vi "Format CSV.vi"(8 "error in (no error)":errorcluster, 9 "delimiter":string=",", 10 "CSV File Input":path, 11 "Original CSV Format":enum16{"Format A", "Format B"}(ring)) -> (0 "error out":errorcluster, 1 "Parcel Length":i32[](array[numeric]), 2 "All Terminal Data":T1(array[cluster]))   [LabVIEW 2017] (continued)
"34:43.4", "34:43.4", "34:43.4", "34:43.5", "34:43.5", "34:43.5", "34:43.6", "34:43.6", "34:43.6", "34:43.7", "34:43.7", "34:43.7", "34:43.8", "34:43.8", "34:43.8", "34:43.9", "34:43.9", "34:43.9", "34:44.0", "34:44.0", "34:44.0", "34:44.1", "34:44.1", "34:44.1", "34:44.2", "34:44.2", "34:44.2", "34:44.3", "34:44.3", "34:44.3", "34:44.4", "34:44.4", "34:44.4", "34:44.5", "34:44.5", "34:44.5", "34:44.6", "34:44.6", "34:44.6", "34:44.7", "34:44.7", "34:44.7", "34:44.8", "34:44.8", "34:44.8", "34:44.9", "34:44.9", "34:44.9", "34:45.0", "34:45.0", "34:45.0", "34:45.1", "34:45.1", "34:45.1", "34:45.2", "34:45.2", "34:45.2", "34:45.3", "34:45.3", "34:45.3", "34:45.4", "34:45.4", "34:45.4", "34:45.5", "34:45.5", "34:45.5", "34:45.6", "34:45.6", "34:45.6", "34:45.7", "34:45.7", "34:45.7", "34:45.8", "34:45.8", "34:45.8", "34:45.9", "34:45.9", "34:45.9", "34:46.0", "34:46.0", "34:46.0", "34:46.1", "34:46.1", "34:46.1", "34:46.2", "34:46.2", "34:46.2", "34:46.3", "34:46.3", "34:46.3", "34:46.4", "34:46.4", "34:46.4", "34:46.5", "34:46.5", "34:46.5", "34:46.6", "34:46.6", "34:46.6", "34:46.7", "34:46.7", "34:46.7", "34:46.8", "34:46.8", "34:46.8", "34:46.9", "34:46.9", "34:46.9", "34:47.0", "34:47.0", "34:47.0", "34:47.1", "34:47.1", "34:47.1", "34:47.2", "34:47.2", "34:47.2", "34:47.3", "34:47.3", "34:47.3", "34:47.4", "34:47.4", "34:47.4", "34:47.5", "34:47.5", "34:47.5", "34:47.6", "34:47.6", "34:47.6", "34:47.7", "34:47.7", "34:47.7", "34:47.8", "34:47.8", "34:47.8", "34:47.9", "34:47.9", "34:47.9", "34:48.0", "34:48.0", "34:48.0", "34:48.1", "34:48.1", "34:48.1", "34:48.2", "34:48.2", "34:48.2", "34:48.3", "34:48.3", "34:48.3", "34:48.4", "34:48.4", "34:48.4", "34:48.5", "34:48.5", "34:48.5", "34:48.6", "34:48.6", "34:48.6", "34:48.7", "34:48.7", "34:48.7", "34:48.8", "34:48.8", "34:48.8", "34:48.9", "34:48.9", "34:48.9", "34:49.0", "34:49.0", "34:49.0", "34:49.1", "34:49.1", "34:49.1", "34:49.2", "34:49.2", "34:49.2", "34:49.3", "34:49.3", "34:49.3", "34:49.4", "34:49.4", "34:49.4", "34:49.5", "34:49.5", "34:49.5", "34:49.6", "34:49.6", "34:49.6", "34:49.7", "34:49.7", "34:49.7", "34:49.8", "34:49.8", "34:49.8", "34:49.9", "34:49.9", "34:49.9", "34:50.0", "34:50.0", "34:50.0", "34:50.1", "34:50.1", "34:50.1", "34:50.2", "34:50.2", "34:50.2", "34:50.3", "34:50.3", "34:50.3", "34:50.4", "34:50.4", "34:50.4", "34:50.5", "34:50.5", "34:50.5", "34:50.6", "34:50.6", "34:50.6", "34:50.7", "34:50.7", "34:50.7", "34:50.8", "34:50.8", "34:50.8", "34:50.9", "34:50.9", "34:50.9", "34:51.0", "34:51.0", "34:51.0", "34:51.1", "34:51.1", "34:51.1", "34:51.2", "34:51.2", "34:51.2", "34:51.3", "34:51.3", "34:51.3", "34:51.4", "34:51.4", "34:51.4", "34:51.5", "34:51.5", "34:51.5", "34:51.6", "34:51.6", "34:51.6", "34:51.7", "34:51.7", "34:51.7", "34:51.8", "34:51.8", "34:51.8", "34:51.9", "34:51.9", "34:51.9", "34:52.0", "34:52.0", "34:52.0", "34:52.1", "34:52.1", "34:52.1", "34:52.2", "34:52.2", "34:52.2", "34:52.3", "34:52.3", "34:52.3", "34:52.4", "34:52.4", "34:52.4", "34:52.5", "34:52.5", "34:52.5", "34:52.6", "34:52.6", "34:52.6", "34:52.7", "34:52.7", "34:52.7", "34:52.8", "34:52.8", "34:52.8", "34:52.9", "34:52.9", "34:52.9", "34:53.0", "34:53.0", "34:53.0", "34:53.1", "34:53.1", "34:53.1", "34:53.2", "34:53.2", "34:53.2", "34:53.3", "34:53.3", "34:53.3", "34:53.4", "34:53.4", "34:53.4", "34:53.5", "34:53.5", "34:53.5", "34:53.6", "34:53.6", "34:53.6", "34:53.7", "34:53.7", "34:53.7", "34:53.8", "34:53.8", "34:53.8", "34:53.9", "34:53.9", "34:53.9", "34:54.0", "34:54.0", "34:54.0", "34:54.1", "34:54.1", "34:54.1", "34:54.2", "34:54.2", "34:54.2", "34:54.3", "34:54.3", "34:54.3", "34:54.4", "34:54.4", "34:54.4", "34:54.5", "34:54.5", "34:54.5", "34:54.6", "34:54.6", "34:54.6", "34:54.7", "34:54.7", "34:54.7", "34:54.8", "34:54.8", "34:54.8", "34:54.9", "34:54.9", "34:54.9", "34:55.0", "34:55.0", "34:55.0", "34:55.1", "34:55.1", "34:55.1", "34:55.2", "34:55.2", "34:55.2", "34:55.3", "34:55.3", "34:55.3", "34:55.4", "34:55.4", "34:55.4", "34:55.5", "34:55.5", "34:55.5", "34:55.6", "34:55.6", "34:55.6", "34:55.7", "34:55.7", "34:55.7", "34:55.8", "34:55.8", "34:55.8", "34:55.9", "34:55.9", "34:55.9", "34:56.0", "34:56.0", "34:56.0", "34:56.1", "34:56.1", "34:56.1", "34:56.2", "34:56.2", "34:56.2", "34:56.3", "34:56.3", "34:56.3", "34:56.4", "34:56.4", "34:56.4", "34:56.5", "34:56.5", "34:56.5", "34:56.6", "34:56.6", "34:56.6", "34:56.7", "34:56.7", "34:56.7", "34:56.8", "34:56.8", "34:56.8", "34:56.9", "34:56.9", "34:56.9", "34:57.0", "34:57.0", "34:57.0", "34:57.1", "34:57.1", "34:57.1", "34:57.2", "34:57.2", "34:57.2", "34:57.3", "34:57.3", "34:57.3", "34:57.4", "34:57.4", "34:57.4", "34:57.5", "34:57.5", "34:57.5", "34:57.6", "34:57.6", "34:57.6", "34:57.7", "34:57.7", "34:57.7", "34:57.8", "34:57.8", "34:57.8", "34:57.9", "34:57.9", "34:57.9", "34:58.0", "34:58.0", "34:58.0", "34:58.1", "34:58.1", "34:58.1", "34:58.2", "34:58.2", "34:58.2", "34:58.3", "34:58.3", "34:58.3", "34:58.4", "34:58.4", "34:58.4", "34:58.5", "34:58.5", "34:58.5", "34:58.6", "34:58.6", "34:58.6", "34:58.7", "34:58.7", "34:58.7", "34:58.8", "34:58.8", "34:58.8", "34:58.9", "34:58.9", "34:58.9", "34:59.0", "34:59.0", "34:59.0", "34:59.1", "34:59.1", "34:59.1", "34:59.2", "34:59.2", "34:59.2", "34:59.3", "34:59.3", "34:59.3", "34:59.4", "34:59.4", "34:59.4", "34:59.5", "34:59.5", "34:59.5", "34:59.6", "34:59.6", "34:59.6", "34:59.7", "34:59.7", "34:59.7", "34:59.8", "34:59.8", "34:59.8", "34:59.9", "34:59.9", "34:59.9", "35:00.0", "35:00.0", "35:00.0", "35:00.1", "35:00.1", "35:00.1", "35:00.2", "35:00.2", "35:00.2", "35:00.3", "35:00.3", "35:00.3", "35:00.4", "35:00.4", "35:00.4", "35:00.5", "35:00.5", "35:00.5", "35:00.6", "35:00.6", "35:00.6", "35:00.7", "35:00.7", "35:00.7", "35:00.8", "35:00.8", "35:00.8", "35:00.9", "35:00.9", "35:00.9", "35:01.0", "35:01.0", "35:01.0", "35:01.1", "35:01.1", "35:01.1", "35:01.2", "35:01.2", "35:01.2", "35:01.3", "35:01.3", "35:01.3", "35:01.4", "35:01.4", "35:01.4", "35:01.5", "35:01.5", "35:01.5", "35:01.6", "35:01.6", "35:01.6", "35:01.7", "35:01.7", "35:01.7", "35:01.8", "35:01.8", "35:01.8", "35:01.9", "35:01.9", "35:01.9", "35:02.0", "35:02.0", "35:02.0", "35:02.1", "35:02.1", "35:02.1", "35:02.2", "35:02.2", "35:02.2", "35:02.3", "35:02.3", "35:02.3", "35:02.4", "35:02.4", "35:02.4", "35:02.5", "35:02.5", "35:02.5", "35:02.6", "35:02.6", "35:02.6", "35:02.7", "35:02.7", "35:02.7", "35:02.8", "35:02.8", "35:02.8", "35:02.9", "35:02.9", "35:02.9", "35:03.0", "35:03.0", "35:03.0", "35:03.1", "35:03.1", "35:03.1", "35:03.2", "35:03.2", "35:03.2", "35:03.3", "35:03.3", "35:03.3", "35:03.4", "35:03.4", "35:03.4", "35:03.5", "35:03.5", "35:03.5", "35:03.6", "35:03.6", "35:03.6", "35:03.7", "35:03.7", "35:03.7", "35:03.8", "35:03.8", "35:03.8", "35:03.9", "35:03.9", "35:03.9", "35:04.0", "35:04.0", "35:04.0", "35:04.1", "35:04.1", "35:04.1", "35:04.2", "35:04.2", "35:04.2", "35:04.3", "35:04.3", "35:04.3", "35:04.4", "35:04.4", "35:04.4", "35:04.5", "35:04.5", "35:04.5", "35:04.6", "35:04.6", "35:04.6", "35:04.7", "35:04.7", "35:04.7", "35:04.8", "35:04.8", "35:04.8", "35:04.9", "35:04.9", "35:04.9", "35:05.0", "35:05.0", "35:05.0", "35:05.1", "35:05.1", "35:05.1", "35:05.2", "35:05.2", "35:05.2", "35:05.3", "35:05.3", "35:05.3", "35:05.4", "35:05.4", "35:05.4", "35:05.5", "35:05.5", "35:05.5", "35:05.6", "35:05.6", "35:05.6", "35:05.7", "35:05.7", "35:05.7", "35:05.8", "35:05.8", "35:05.8", "35:05.9", "35:05.9", "35:05.9", "35:06.0", "35:06.0", "35:06.0", "35:06.1", "35:06.1", "35:06.1", "35:06.2", "35:06.2", "35:06.2", "35:06.3", "35:06.3", "35:06.3", "35:06.4", "35:06.4", "35:06.4", "35:06.5", "35:06.5", "35:06.5", "35:06.6", "35:06.6", "35:06.6", "35:06.7", "35:06.7", "35:06.7", "35:06.8", "35:06.8", "35:06.8", "35:06.9", "35:06.9", "35:06.9", "35:07.0", "35:07.0", "35:07.0", "35:07.1", "35:07.1", "35:07.1", "35:07.2", "35:07.2", "35:07.2", "35:07.3", "35:07.3", "35:07.3", "35:07.4", "35:07.4", "35:07.4", "35:07.5", "35:07.5", "35:07.5", "35:07.6", "35:07.6", "35:07.6", "35:07.7", "35:07.7", "35:07.7", "35:07.8", "35:07.8", "35:07.8", "35:07.9", "35:07.9", "35:07.9", "35:08.0", "35:08.0", "35:08.0", "35:08.1", "35:08.1", "35:08.1", "35:08.2", "35:08.2", "35:08.2", "35:08.3", "35:08.3", "35:08.3", "35:08.4", "35:08.4", "35:08.4", "35:08.5", "35:08.5", "35:08.5", "35:08.6", "35:08.6", "35:08.6", "35:08.7", "35:08.7", "35:08.7", "35:08.8", "35:08.8", "35:08.8", "35:08.9", "35:08.9", "35:08.9", "35:09.0", "35:09.0", "35:09.0", "35:09.1", "35:09.1", "35:09.1", "35:09.2", "35:09.2", "35:09.2", "35:09.3", "35:09.3", "35:09.3", "35:09.4", "35:09.4", "35:09.4", "35:09.5", "35:09.5", "35:09.5", "35:09.6", "35:09.6", "35:09.6", "35:09.7", "35:09.7", "35:09.7", "35:09.8", "35:09.8", "35:09.8", "35:09.9", "35:09.9", "35:09.9", "35:10.0", "35:10.0", "35:10.0", "35:10.1", "35:10.1", "35:10.1", "35:10.2", "35:10.2", "35:10.2", "35:10.3", "35:10.3", "35:10.3", "35:10.4", "35:10.4", "35:10.4", "35:10.5", "35:10.5", "35:10.5", "35:10.6", "35:10.6", "35:10.6", "35:10.7", "35:10.7", "35:10.7", "35:10.8", "35:10.8", "35:10.8", "35:10.9", "35:10.9", "35:10.9", "35:11.0", "35:11.0", "35:11.0", "35:11.1", "35:11.1", "35:11.1", "35:11.2", "35:11.2", "35:11.2", "35:11.3", "35:11.3", "35:11.3", "35:11.4", "35:11.4", "35:11.4", "35:11.5", "35:11.5", "35:11.5", "35:11.6", "35:11.6", "35:11.6", "35:11.7", "35:11.7", "35:11.7", "35:11.8", "35:11.8", "35:11.8", "35:11.9", "35:11.9", "35:11.9", "35:12.0", "35:12.0", "35:12.0", "35:12.1", "35:12.1", "35:12.1", "35:12.2", "35:12.2", "35:12.2", "35:12.3", "35:12.3", "35:12.3", "35:12.4", "35:12.4", "35:12.4", "35:12.5", "35:12.5", "35:12.5", "35:12.6", "35:12.6", "35:12.6", "35:12.7", "35:12.7", "35:12.7", "35:12.8", "35:12.8", "35:12.8", "35:12.9", "35:12.9", "35:12.9", "35:13.0", "35:13.0", "35:13.0", "35:13.1", "35:13.1", "35:13.1", "35:13.2", "35:13.2", "35:13.2", "35:13.3", "35:13.3", "35:13.3", "35:13.4", "35:13.4", "35:13.4", "35:13.5", "35:13.5", "35:13.5", "35:13.6", "35:13.6", "35:13.6", "35:13.7", "35:13.7", "35:13.7", "35:13.8", "35:13.8", "35:13.8", "35:13.9", "35:13.9", "35:13.9", "35:14.0", "35:14.0", "35:14.0", "35:14.1", "35:14.1", "35:14.1", "35:14.2", "35:14.2", "35:14.2", "35:14.3", "35:14.3", "35:14.3", "35:14.4", "35:14.4", "35:14.4", "35:14.5", "35:14.5", "35:14.5", "35:14.6", "35:14.6", "35:14.6", "35:14.7", "35:14.7", "35:14.7", "35:14.8", "35:14.8", "35:14.8", "35:14.9", "35:14.9", "35:14.9", "35:15.0", "35:15.0", "35:15.0", "35:15.1", "35:15.1", "35:15.1", "35:15.2", "35:15.2", "35:15.2", "35:15.3", "35:15.3", "35:15.3", "35:15.4", "35:15.4", "35:15.4", "35:15.5", "35:15.5", "35:15.5", "35:15.6", "35:15.6", "35:15.6", "35:15.7", "35:15.7", "35:15.7", "35:15.8", "35:15.8", "35:15.8", "35:15.9", "35:15.9", "35:15.9", "35:16.0", "35:16.0", "35:16.0", "35:16.1", "35:16.1", "35:16.1", "35:16.2", "35:16.2", "35:16.2", "35:16.3", "35:16.3", "35:16.3", "35:16.4", "35:16.4", "35:16.4", "35:16.5", "35:16.5", "35:16.5", "35:16.6", "35:16.6", "35:16.6", "35:16.7", "35:16.7", "35:16.7", "35:16.8", "35:16.8", "35:16.8", "35:16.9", "35:16.9", "35:16.9", "35:17.0", "35:17.0", "35:17.0", "35:17.1", "35:17.1", "35:17.1", "35:17.2", "35:17.2", "35:17.2", "35:17.3", "35:17.3", "35:17.3", "35:17.4", "35:17.4", "35:17.4", "35:17.5", "35:17.5", "35:17.5", "35:17.6", "35:17.6", "35:17.6", "35:17.7", "35:17.7", "35:17.7", "35:17.8", "35:17.8", "35:17.8", "35:17.9", "35:17.9", "35:17.9", "35:18.0", "35:18.0", "35:18.0", "35:18.1", "35:18.1", "35:18.1", "35:18.2", "35:18.2", "35:18.2", "35:18.3", "35:18.3", "35:18.3", "35:18.4", "35:18.4", "35:18.4", "35:18.5", "35:18.5", "35:18.5", "35:18.6", "35:18.6", "35:18.6", "35:18.7", "35:18.7", "35:18.7", "35:18.8", "35:18.8", "35:18.8", "35:18.9", "35:18.9", "35:18.9", "35:19.0", "35:19.0", "35:19.0", "35:19.1", "35:19.1", "35:19.1", "35:19.2", "35:19.2", "35:19.2", "35:19.3", "35:19.3", "35:19.3", "35:19.4", "35:19.4", "35:19.4", "35:19.5", "35:19.5", "35:19.5", "35:19.6", "35:19.6", "35:19.6", "35:19.7", "35:19.7", "35:19.7", "35:19.8", "35:19.8", "35:19.8", "35:19.9", "35:19.9", "35:19.9", "35:20.0", "35:20.0", "35:20.0", "35:20.1", "35:20.1", "35:20.1", "35:20.2", "35:20.2", "35:20.2", "35:20.3", "35:20.3", "35:20.3", "35:20.4", "35:20.4", "35:20.4", "35:20.5", "35:20.5", "35:20.5", "35:20.6", "35:20.6", "35:20.6", "35:20.7", "35:20.7", "35:20.7", "35:20.8", "35:20.8", "35:20.8", "35:20.9", "35:20.9", "35:20.9", "35:21.0", "35:21.0", "35:21.0", "35:21.1", "35:21.1", "35:21.1", "35:21.2", "35:21.2", "35:21.2", "35:21.3", "35:21.3", "35:21.3", "35:21.4", "35:21.4", "35:21.4", "35:21.5", "35:21.5", "35:21.5", "35:21.6", "35:21.6", "35:21.6", "35:21.7", "35:21.7", "35:21.7", "35:21.8", "35:21.8", "35:21.8", "35:21.9", "35:21.9", "35:21.9", "35:22.0", "35:22.0", "35:22.0", "35:22.1", "35:22.1", "35:22.1", "35:22.2", "35:22.2", "35:22.2", "35:22.3", "35:22.3", "35:22.3", "35:22.4", "35:22.4", "35:22.4", "35:22.5", "35:22.5", "35:22.5", "35:22.6", "35:22.6", "35:22.6", "35:22.7", "35:22.7", "35:22.7", "35:22.8", "35:22.8", "35:22.8", "35:22.9", "35:22.9", "35:22.9", "35:23.0", "35:23.0", "35:23.0", "35:23.1", "35:23.1", "35:23.1", "35:23.2", "35:23.2", "35:23.2", "35:23.3", "35:23.3", "35:23.3", "35:23.4", "35:23.4", "35:23.4", "35:23.5", "35:23.5", "35:23.5", "35:23.6", "35:23.6", "35:23.6", "35:23.7", "35:23.7", "35:23.7", "35:23.8", "35:23.8", "35:23.8", "35:23.9", "35:23.9", "35:23.9", "35:24.0", "35:24.0", "35:24.0", "35:24.1", "35:24.1", "35:24.1", "35:24.2", "35:24.2", "35:24.2", "35:24.3", "35:24.3", "35:24.3", "35:24.4", "35:24.4", "35:24.4", "35:24.5", "35:24.5", "35:24.5", "35:24.6", "35:24.6", "35:24.6", "35:24.7", "35:24.7", "35:24.7", "35:24.8", "35:24.8", "35:24.8", "35:24.9", "35:24.9", "35:24.9", "35:25.0", "35:25.0", "35:25.0", "35:25.1", "35:25.1", "35:25.1", "35:25.2", "35:25.2", "35:25.2", "35:25.3", "35:25.3", "35:25.3", "35:25.4", "35:25.4", "35:25.4", "35:25.5", "35:25.5", "35:25.5", "35:25.6", "35:25.6", "35:25.6", "35:25.7", "35:25.7", "35:25.7", "35:25.8", "35:25.8", "35:25.8", "35:25.9", "35:25.9", "35:25.9", "35:26.0", "35:26.0", "35:26.0", "35:26.1", "35:26.1", "35:26.1", "35:26.2", "35:26.2", "35:26.2", "35:26.3", "35:26.3", "35:26.3", "35:26.4", "35:26.4", "35:26.4", "35:26.5", "35:26.5", "35:26.5", "35:26.6", "35:26.6", "35:26.6", "35:26.7", "35:26.7", "35:26.7", "35:26.8", "35:26.8", "35:26.8", "35:26.9", "35:26.9", "35:26.9", "35:27.0", "35:27.0", "35:27.0", "35:27.1", "35:27.1", "35:27.1", "35:27.2", "35:27.2", "35:27.2", "35:27.3", "35:27.3", "35:27.3", "35:27.4", "35:27.4", "35:27.4", "35:27.5", "35:27.5", "35:27.5", "35:27.6", "35:27.6", "35:27.6", "35:27.7", "35:27.7", "35:27.7", "35:27.8", "35:27.8", "35:27.8", "35:27.9", "35:27.9", "35:27.9", "35:28.0", "35:28.0", "35:28.0", "35:28.1", "35:28.1", "35:28.1", "35:28.2", "35:28.2", "35:28.2", "35:28.3", "35:28.3", "35:28.3", "35:28.4", "35:28.4", "35:28.4", "35:28.5", "35:28.5", "35:28.5", "35:28.6", "35:28.6", "35:28.6", "35:28.7", "35:28.7", "35:28.7", "35:28.8", "35:28.8", "35:28.8", "35:28.9", "35:28.9", "35:28.9", "35:29.0", "35:29.0", "35:29.0", "35:29.1", "35:29.1", "35:29.1", "35:29.2", "35:29.2", "35:29.2", "35:29.3", "35:29.3", "35:29.3", "35:29.4", "35:29.4", "35:29.4", "35:29.5", "35:29.5", "35:29.5", "35:29.6", "35:29.6", "35:29.6", "35:29.7", "35:29.7", "35:29.7", "35:29.8", "35:29.8", "35:29.8", "35:29.9", "35:29.9", "35:29.9", "35:30.0", "35:30.0", "35:30.0", "35:30.1", "35:30.1", "35:30.1", "35:30.2", "35:30.2", "35:30.2", "35:30.3", "35:30.3", "35:30.3", "35:30.4", "35:30.4", "35:30.4", "35:30.5", "35:30.5", "35:30.5", "35:30.6", "35:30.6", "35:30.6", "35:30.7", "35:30.7", "35:30.7", "35:30.8", "35:30.8", "35:30.8", "35:30.9", "35:30.9", "35:30.9", "35:31.0", "35:31.0", "35:31.0", "35:31.1", "35:31.1", "35:31.1", "35:31.2", "35:31.2", "35:31.2", "35:31.3", "35:31.3", "35:31.3", "35:31.4", "35:31.4", "35:31.4", "35:31.5", "35:31.5", "35:31.5", "35:31.6", "35:31.6", "35:31.6", "35:31.7", "35:31.7", "35:31.7", "35:31.8", "35:31.8", "35:31.8", "35:31.9", "35:31.9", "35:31.9", "35:32.0", "35:32.0", "35:32.0", "35:32.1", "35:32.1", "35:32.1", "35:32.2", "35:32.2", "35:32.2", "35:32.3", "35:32.3", "35:32.3", "35:32.4", "35:32.4", "35:32.4", "35:32.5", "35:32.5", "35:32.5", "35:32.6", "35:32.6", "35:32.6", "35:32.7", "35:32.7", "35:32.7", "35:32.8", "35:32.8", "35:32.8", "35:32.9", "35:32.9", "35:32.9", "35:33.0", "35:33.0", "35:33.0", "35:33.1", "35:33.1", "35:33.1", "35:33.2", "35:33.2", "35:33.2", "35:33.3", "35:33.3", "35:33.3", "35:33.4", "35:33.4", "35:33.4", "35:33.5", "35:33.5", "35:33.5", "35:33.6", "35:33.6", "35:33.6", "35:33.7", "35:33.7", "35:33.7", "35:33.8", "35:33.8", "35:33.8", "35:33.9", "35:33.9", "35:33.9", "35:34.0", "35:34.0", "35:34.0", "35:34.1", "35:34.1", "35:34.1", "35:34.2", "35:34.2", "35:34.2", "35:34.3", "35:34.3", "35:34.3", "35:34.4", "35:34.4", "35:34.4", "35:34.5", "35:34.5", "35:34.5", "35:34.6", "35:34.6", "35:34.6", "35:34.7", "35:34.7", "35:34.7", "35:34.8", "35:34.8", "35:34.8", "35:34.9", "35:34.9", "35:34.9", "35:35.0", "35:35.0", "35:35.0", "35:35.1", "35:35.1", "35:35.1", "35:35.2", "35:35.2", "35:35.2", "35:35.3", "35:35.3", "35:35.3", "35:35.4", "35:35.4", "35:35.4", "35:35.5", "35:35.5", "35:35.5", "35:35.6", "35:35.6", "35:35.6", "35:35.7", "35:35.7", "35:35.7", "35:35.8", "35:35.8", "35:35.8", "35:35.9", "35:35.9", "35:35.9", "35:36.0", "35:36.0", "35:36.0", "35:36.1", "35:36.1", "35:36.1", "35:36.2", "35:36.2", "35:36.2", "35:36.3", "35:36.3", "35:36.3", "35:36.4", "35:36.4", "35:36.4", "35:36.5", "35:36.5", "35:36.5", "35:36.6", "35:36.6", "35:36.6", "35:36.7", "35:36.7", "35:36.7", "35:36.8", "35:36.8", "35:36.8", "35:36.9", "35:36.9", "35:36.9", "35:37.0", "35:37.0", "35:37.0", "35:37.1", "35:37.1", "35:37.1", "35:37.2", "35:37.2", "35:37.2", "35:37.3", "35:37.3", "35:37.3", "35:37.4", "35:37.4", "35:37.4", "35:37.5", "35:37.5", "35:37.5", "35:37.6", "35:37.6", "35:37.6", "35:37.7", "35:37.7", "35:37.7", "35:37.8", "35:37.8", "35:37.8", "35:37.9", "35:37.9", "35:37.9", "35:38.0", "35:38.0", "35:38.0", "35:38.1", "35:38.1", "35:38.1", "35:38.2", "35:38.2", "35:38.2", "35:38.3", "35:38.3", "35:38.3", "35:38.4", "35:38.4", "35:38.4", "35:38.5", "35:38.5", "35:38.5", "35:38.6", "35:38.6", "35:38.6", "35:38.7", "35:38.7", "35:38.7", "35:38.8", "35:38.8", "35:38.8", "35:38.9", "35:38.9", "35:38.9", "35:39.0", "35:39.0", "35:39.0", "35:39.1", "35:39.1", "35:39.1", "35:39.2", "35:39.2", "35:39.2", "35:39.3", "35:39.3", "35:39.3", "35:39.4", "35:39.4", "35:39.4", "35:39.5", "35:39.5", "35:39.5", "35:39.6", "35:39.6", "35:39.6", "35:39.7", "35:39.7", "35:39.7", "35:39.8", "35:39.8", "35:39.8", "35:39.9", "35:39.9", "35:39.9", "35:40.0", "35:40.0", "35:40.0", "35:40.1", "35:40.1", "35:40.1", "35:40.2", "35:40.2", "35:40.2", "35:40.3", "35:40.3", "35:40.3", "35:40.4", "35:40.4", "35:40.4", "35:40.5", "35:40.5", "35:40.5", "35:40.6", "35:40.6", "35:40.6", "35:40.7", "35:40.7", "35:40.7", "35:40.8", "35:40.8", "35:40.8", "35:40.9", "35:40.9", "35:40.9", "35:41.0", "35:41.0", "35:41.0", "35:41.1", "35:41.1", "35:41.1", "35:41.2", "35:41.2", "35:41.2", "35:41.3", "35:41.3", "35:41.3", "35:41.4", "35:41.4", "35:41.4", "35:41.5", "35:41.5", "35:41.5", "35:41.6", "35:41.6", "35:41.6", "35:41.7", "35:41.7", "35:41.7", "35:41.8", "35:41.8", "35:41.8", "35:41.9", "35:41.9", "35:41.9", "35:42.0", "35:42.0", "35:42.0", "35:42.1", "35:42.1", "35:42.1", "35:42.2", "35:42.2", "35:42.2", "35:42.3", "35:42.3", "35:42.3", "35:42.4", "35:42.4", "35:42.4", "35:42.5", "35:42.5", "35:42.5", "35:42.6", "35:42.6", "35:42.6", "35:42.7", "35:42.7", "35:42.7", "35:42.8", "35:42.8", "35:42.8", "35:42.9", "35:42.9", "35:42.9", "35:43.0", "35:43.0", "35:43.0", "35:43.1", "35:43.1", "35:43.1", "35:43.2", "35:43.2", "35:43.2", "35:43.3", "35:43.3", "35:43.3", "35:43.4", "35:43.4", "35:43.4", "35:43.5", "35:43.5", "35:43.5", "35:43.6", "35:43.6", "35:43.6", "35:43.7", "35:43.7", "35:43.7", "35:43.8", "35:43.8", "35:43.8", "35:43.9", "35:43.9", "35:43.9", "35:44.0", "35:44.0", "35:44.0", "35:44.1", "35:44.1", "35:44.1", "35:44.2", "35:44.2", "35:44.2", "35:44.3", "35:44.3", "35:44.3", "35:44.4", "35:44.4", "35:44.4", "35:44.5", "35:44.5", "35:44.5", "35:44.6", "35:44.6", "35:44.6", "35:44.7", "35:44.7", "35:44.7", "35:44.8", "35:44.8", "35:44.8", "35:44.9", "35:44.9", "35:44.9", "35:45.0", "35:45.0", "35:45.0", "35:45.1", "35:45.1", "35:45.1", "35:45.2", "35:45.2", "35:45.2", "35:45.3", "35:45.3", "35:45.3", "35:45.4", "35:45.4", "35:45.4", "35:45.5", "35:45.5", "35:45.5", "35:45.6", "35:45.6", "35:45.6", "35:45.7", "35:45.7", "35:45.7", "35:45.8", "35:45.8", "35:45.8", "35:45.9", "35:45.9", "35:45.9", "35:46.0", "35:46.0", "35:46.0", "35:46.1", "35:46.1", "35:46.1", "35:46.2", "35:46.2", "35:46.2", "35:46.3", "35:46.3", "35:46.3", "35:46.4", "35:46.4", "35:46.4", "35:46.5", "35:46.5", "35:46.5", "35:46.6", "35:46.6", "35:46.6", "35:46.7", "35:46.7", "35:46.7", "35:46.8", "35:46.8", "35:46.8", "35:46.9", "35:46.9", "35:46.9", "35:47.0", "35:47.0", "35:47.0", "35:47.1", "35:47.1", "35:47.1", "35:47.2", "35:47.2", "35:47.2", "35:47.3", "35:47.3", "35:47.3", "35:47.4", "35:47.4", "35:47.4", "35:47.5", "35:47.5", "35:47.5", "35:47.6", "35:47.6", "35:47.6", "35:47.7", "35:47.7", "35:47.7", "35:47.8", "35:47.8", "35:47.8", "35:47.9", "35:47.9", "35:47.9", "35:48.0", "35:48.0", "35:48.0", "35:48.1", "35:48.1", "35:48.1", "35:48.2", "35:48.2", "35:48.2", "35:48.3", "35:48.3", "35:48.3", "35:48.4", "35:48.4", "35:48.4", "35:48.5", "35:48.5", "35:48.5", "35:48.6", "35:48.6", "35:48.6", "35:48.7", "35:48.7", "35:48.7", "35:48.8", "35:48.8", "35:48.8", "35:48.9", "35:48.9", "35:48.9", "35:49.0", "35:49.0", "35:49.0", "35:49.1", "35:49.1", "35:49.1", "35:49.2", "35:49.2", "35:49.2", "35:49.3", "35:49.3", "35:49.3", "35:49.4", "35:49.4", "35:49.4", "35:49.5", "35:49.5", "35:49.5", "35:49.6", "35:49.6", "35:49.6", "35:49.7", "35:49.7", "35:49.7", "35:49.8", "35:49.8", "35:49.8", "35:49.9", "35:49.9", "35:49.9", "35:50.0", "35:50.0", "35:50.0", "35:50.1", "35:50.1", "35:50.1", "35:50.2", "35:50.2", "35:50.2", "35:50.3", "35:50.3", "35:50.3", "35:50.4", "35:50.4", "35:50.4", "35:50.5", "35:50.5", "35:50.5", "35:50.6", "35:50.6", "35:50.6", "35:50.7", "35:50.7", "35:50.7", "35:50.8", "35:50.8", "35:50.8", "35:50.9", "35:50.9", "35:50.9", "35:51.0", "35:51.0", "35:51.0", "35:51.1", "35:51.1", "35:51.1", "35:51.2", "35:51.2", "35:51.2", "35:51.3", "35:51.3", "35:51.3", "35:51.4", "35:51.4", "35:51.4", "35:51.5", "35:51.5", "35:51.5", "35:51.6", "35:51.6", "35:51.6", "35:51.7", "35:51.7", "35:51.7", "35:51.8", "35:51.8", "35:51.8", "35:51.9", "35:51.9", "35:51.9", "35:52.0", "35:52.0", "35:52.0", "35:52.1", "35:52.1", "35:52.1", "35:52.2", "35:52.2", "35:52.2", "35:52.3", "35:52.3", "35:52.3", "35:52.4", "35:52.4", "35:52.4", "35:52.5", "35:52.5", "35:52.5", "35:52.6", "35:52.6", "35:52.6", "35:52.7", "35:52.7", "35:52.7", "35:52.8", "35:52.8", "35:52.8", "35:52.9", "35:52.9", "35:52.9", "35:53.0", "35:53.0", "35:53.0", "35:53.1", "35:53.1", "35:53.1", "35:53.2", "35:53.2", "35:53.2", "35:53.3", "35:53.3", "35:53.3", "35:53.4", "35:53.4", "35:53.4", "35:53.5", "35:53.5", "35:53.5", "35:53.6", "35:53.6", "35:53.6", "35:53.7", "35:53.7", "35:53.7", "35:53.8", "35:53.8", "35:53.8", "35:53.9", "35:53.9", "35:53.9", "35:54.0", "35:54.0", "35:54.0", "35:54.1", "35:54.1", "35:54.1", "35:54.2", "35:54.2", "35:54.2", "35:54.3", "35:54.3", "35:54.3", "35:54.4", "35:54.4", "35:54.4", "35:54.5", "35:54.5", "35:54.5", "35:54.6", "35:54.6", "35:54.6", "35:54.7", "35:54.7", "35:54.7", "35:54.8", "35:54.8", "35:54.8", "35:54.9", "35:54.9", "35:54.9", "35:55.0", "35:55.0", "35:55.0", "35:55.1", "35:55.1", "35:55.1", "35:55.2", "35:55.2", "35:55.2", "35:55.3", "35:55.3", "35:55.3", "35:55.4", "35:55.4", "35:55.4", "35:55.5", "35:55.5", "35:55.5", "35:55.6", "35:55.6", "35:55.6", "35:55.7", "35:55.7", "35:55.7", "35:55.8", "35:55.8", "35:55.8", "35:55.9", "35:55.9", "35:55.9", "35:56.0", "35:56.0", "35:56.0", "35:56.1", "35:56.1", "35:56.1", "35:56.2", "35:56.2", "35:56.2", "35:56.3", "35:56.3", "35:56.3", "35:56.4", "35:56.4", "35:56.4", "35:56.5", "35:56.5", "35:56.5", "35:56.6", "35:56.6", "35:56.6", "35:56.7", "35:56.7", "35:56.7", "35:56.8", "35:56.8", "35:56.8", "35:56.9", "35:56.9", "35:56.9", "35:57.0", "35:57.0", "35:57.0", "35:57.1", "35:57.1", "35:57.1", "35:57.2", "35:57.2", "35:57.2", "35:57.3", "35:57.3", "35:57.3", "35:57.4", "35:57.4", "35:57.4", "35:57.5", "35:57.5", "35:57.5", "35:57.6", "35:57.6", "35:57.6", "35:57.7", "35:57.7", "35:57.7", "35:57.8", "35:57.8", "35:57.8", "35:57.9", "35:57.9", "35:57.9", "35:58.0", "35:58.0", "35:58.0", "35:58.1", "35:58.1", "35:58.1", "35:58.2", "35:58.2", "35:58.2", "35:58.3", "35:58.3", "35:58.3", "35:58.4", "35:58.4", "35:58.4", "35:58.5", "35:58.5", "35:58.5", "35:58.6", "35:58.6", "35:58.6", "35:58.7", "35:58.7", "35:58.7", "35:58.8", "35:58.8", "35:58.8", "35:58.9", "35:58.9", "35:58.9", "35:59.0", "35:59.0", "35:59.0", "35:59.1", "35:59.1", "35:59.1", "35:59.2", "35:59.2", "35:59.2", "35:59.3", "35:59.3", "35:59.3", "35:59.4", "35:59.4", "35:59.4", "35:59.5", "35:59.5", "35:59.5", "35:59.6", "35:59.6", "35:59.6", "35:59.7", "35:59.7", "35:59.7", "35:59.8", "35:59.8", "35:59.8", "35:59.9", "35:59.9", "35:59.9", "36:00.0", "36:00.0", "36:00.0", "36:00.1", "36:00.1", "36:00.1", "36:00.2", "36:00.2", "36:00.2", "36:00.3", "36:00.3", "36:00.3", "36:00.4", "36:00.4", "36:00.4", "36:00.5", "36:00.5", "36:00.5", "36:00.6", "36:00.6", "36:00.6", "36:00.7", "36:00.7", "36:00.7", "36:00.8", "36:00.8", "36:00.8", "36:00.9", "36:00.9", "36:00.9", "36:01.0", "36:01.0", "36:01.0", "36:01.1", "36:01.1", "36:01.1", "36:01.2", "36:01.2", "36:01.2", "36:01.3", "36:01.3", "36:01.3", "36:01.4", "36:01.4", "36:01.4", "36:01.5", "36:01.5", "36:01.5", "36:01.6", "36:01.6", "36:01.6", "36:01.7", "36:01.7", "36:01.7", "36:01.8", "36:01.8", "36:01.8", "36:01.9", "36:01.9", "36:01.9", "36:02.0", "36:02.0", "36:02.0", "36:02.1", "36:02.1", "36:02.1", "36:02.2", "36:02.2", "36:02.2", "36:02.3", "36:02.3", "36:02.3", "36:02.4", "36:02.4", "36:02.4", "36:02.5", "36:02.5", "36:02.5", "36:02.6", "36:02.6", "36:02.6", "36:02.7", "36:02.7", "36:02.7", "36:02.8", "36:02.8", "36:02.8", "36:02.9", "36:02.9", "36:02.9", "36:03.0", "36:03.0", "36:03.0", "36:03.1", "36:03.1", "36:03.1", "36:03.2", "36:03.2", "36:03.2", "36:03.3", "36:03.3", "36:03.3", "36:03.4", "36:03.4", "36:03.4", "36:03.5", "36:03.5", "36:03.5", "36:03.6", "36:03.6", "36:03.6", "36:03.7", "36:03.7", "36:03.7", "36:03.8", "36:03.8", "36:03.8", "36:03.9", "36:03.9", "36:03.9", "36:04.0", "36:04.0", "36:04.0", "36:04.1", "36:04.1", "36:04.1", "36:04.2", "36:04.2", "36:04.2", "36:04.3", "36:04.3", "36:04.3", "36:04.4", "36:04.4", "36:04.4", "36:04.5", "36:04.5", "36:04.5", "36:04.6", "36:04.6", "36:04.6", "36:04.7", "36:04.7", "36:04.7", "36:04.8", "36:04.8", "36:04.8", "36:04.9", "36:04.9", "36:04.9", "36:05.0", "36:05.0", "36:05.0", "36:05.1", "36:05.1", "36:05.1", "36:05.2", "36:05.2", "36:05.2", "36:05.3", "36:05.3", "36:05.3", "36:05.4", "36:05.4", "36:05.4", "36:05.5", "36:05.5", "36:05.5", "36:05.6", "36:05.6", "36:05.6", "36:05.7", "36:05.7", "36:05.7", "36:05.8", "36:05.8", "36:05.8", "36:05.9", "36:05.9", "36:05.9", "36:06.0", "36:06.0", "36:06.0", "36:06.1", "36:06.1", "36:06.1", "36:06.2", "36:06.2", "36:06.2", "36:06.3", "36:06.3", "36:06.3", "36:06.4", "36:06.4", "36:06.4", "36:06.5", "36:06.5", "36:06.5", "36:06.6", "36:06.6", "36:06.6", "36:06.7", "36:06.7", "36:06.7", "36:06.8", "36:06.8", "36:06.8", "36:06.9", "36:06.9", "36:06.9", "36:07.0", "36:07.0", "36:07.0", "36:07.1", "36:07.1", "36:07.1", "36:07.2", "36:07.2", "36:07.2", "36:07.3", "36:07.3", "36:07.3", "36:07.4", "36:07.4", "36:07.4", "36:07.5", "36:07.5", "36:07.5", "36:07.6", "36:07.6", "36:07.6", "36:07.7", "36:07.7", "36:07.7", "36:07.8", "36:07.8", "36:07.8", "36:07.9", "36:07.9", "36:07.9", "36:08.0", "36:08.0", "36:08.0", "36:08.1", "36:08.1", "36:08.1", "36:08.2", "36:08.2", "36:08.2", "36:08.3", "36:08.3", "36:08.3", "36:08.4", "36:08.4", "36:08.4", "36:08.5", "36:08.5", "36:08.5", "36:08.6", "36:08.6", "36:08.6", "36:08.7", "36:08.7", "36:08.7", "36:08.8", "36:08.8", "36:08.8", "36:08.9", "36:08.9", "36:08.9", "36:09.0", "36:09.0", "36:09.0", "36:09.1", "36:09.1", "36:09.1", "36:09.2", "36:09.2", "36:09.2", "36:09.3", "36:09.3", "36:09.3", "36:09.4", "36:09.4", "36:09.4", "36:09.5", "36:09.5", "36:09.5", "36:09.6", "36:09.6", "36:09.6", "36:09.7", "36:09.7", "36:09.7", "36:09.8", "36:09.8", "36:09.8", "36:09.9", "36:09.9", "36:09.9", "36:10.0", "36:10.0", "36:10.0", "36:10.1", "36:10.1", "36:10.1", "36:10.2", "36:10.2", "36:10.2", "36:10.3", "36:10.3", "36:10.3", "36:10.4", "36:10.4", "36:10.4", "36:10.5", "36:10.5", "36:10.5", "36:10.6", "36:10.6", "36:10.6", "36:10.7", "36:10.7", "36:10.7", "36:10.8", "36:10.8", "36:10.8", "36:10.9", "36:10.9", "36:10.9", "36:11.0", "36:11.0", "36:11.0", "36:11.1", "36:11.1", "36:11.1", "36:11.2", "36:11.2", "36:11.2", "36:11.3", "36:11.3", "36:11.3", "36:11.4", "36:11.4", "36:11.4", "36:11.5", "36:11.5", "36:11.5", "36:11.6", "36:11.6", "36:11.6", "36:11.7", "36:11.7", "36:11.7", "36:11.8", "36:11.8", "36:11.8", "36:11.9", "36:11.9", "36:11.9", "36:12.0", "36:12.0", "36:12.0", "36:12.1", "36:12.1", "36:12.1", "36:12.2", "36:12.2", "36:12.2", "36:12.3", "36:12.3", "36:12.3", "36:12.4", "36:12.4", "36:12.4", "36:12.5", "36:12.5", "36:12.5", "36:12.6", "36:12.6", "36:12.6", "36:12.7", "36:12.7", "36:12.7", "36:12.8", "36:12.8", "36:12.8", "36:12.9", "36:12.9", "36:12.9", "36:13.0", "36:13.0", "36:13.0", "36:13.1", "36:13.1", "36:13.1", "36:13.2", "36:13.2", "36:13.2", "36:13.3", "36:13.3", "36:13.3", "36:13.4", "36:13.4", "36:13.4", "36:13.5", "36:13.5", "36:13.5", "36:13.6", "36:13.6", "36:13.6", "36:13.7", "36:13.7", "36:13.7", "36:13.8", "36:13.8", "36:13.8", "36:13.9", "36:13.9", "36:13.9", "36:14.0", "36:14.0", "36:14.0", "36:14.1", "36:14.1", "36:14.1", "36:14.2", "36:14.2", "36:14.2", "36:14.3", "36:14.3", "36:14.3", "36:14.4", "36:14.4", "36:14.4", "36:14.5", "36:14.5", "36:14.5", "36:14.6", "36:14.6", "36:14.6", "36:14.7", "36:14.7", "36:14.7", "36:14.8", "36:14.8", "36:14.8", "36:14.9", "36:14.9", "36:14.9", "36:15.0", "36:15.0", "36:15.0", "36:15.1", "36:15.1", "36:15.1", "36:15.2", "36:15.2", "36:15.2", "36:15.3", "36:15.3", "36:15.3", "36:15.4", "36:15.4", "36:15.4", "36:15.5", "36:15.5", "36:15.5", "36:15.6", "36:15.6", "36:15.6", "36:15.7", "36:15.7", "36:15.7", "36:15.8", "36:15.8", "36:15.8", "36:15.9", "36:15.9", "36:15.9", "36:16.0", "36:16.0", "36:16.0", "36:16.1", "36:16.1", "36:16.1", "36:16.2", "36:16.2", "36:16.2", "36:16.3", "36:16.3", "36:16.3", "36:16.4", "36:16.4", "36:16.4", "36:16.5", "36:16.5", "36:16.5", "36:16.6", "36:16.6", "36:16.6", "36:16.7", "36:16.7", "36:16.7", "36:16.8", "36:16.8", "36:16.8", "36:16.9", "36:16.9", "36:16.9", "36:17.0", "36:17.0", "36:17.0", "36:17.1", "36:17.1", "36:17.1", "36:17.2", "36:17.2", "36:17.2", "36:17.3", "36:17.3", "36:17.3", "36:17.4", "36:17.4", "36:17.4", "36:17.5", "36:17.5", "36:17.5", "36:17.6", "36:17.6", "36:17.6", "36:17.7", "36:17.7", "36:17.7", "36:17.8", "36:17.8", "36:17.8", "36:17.9", "36:17.9", "36:17.9", "36:18.0", "36:18.0", "36:18.0", "36:18.1", "36:18.1", "36:18.1", "36:18.2", "36:18.2", "36:18.2", "36:18.3", "36:18.3", "36:18.3", "36:18.4", "36:18.4", "36:18.4", "36:18.5", "36:18.5", "36:18.5", "36:18.6", "36:18.6", "36:18.6", "36:18.7", "36:18.7", "36:18.7", "36:18.8", "36:18.8", "36:18.8", "36:18.9", "36:18.9", "36:18.9", "36:19.0", "36:19.0", "36:19.0", "36:19.1", "36:19.1", "36:19.1", "36:19.2", "36:19.2", "36:19.2", "36:19.3", "36:19.3", "36:19.3", "36:19.4", "36:19.4", "36:19.4", "36:19.5", "36:19.5", "36:19.5", "36:19.6", "36:19.6", "36:19.6", "36:19.7", "36:19.7", "36:19.7", "36:19.8", "36:19.8", "36:19.8", "36:19.9", "36:19.9", "36:19.9", "36:20.0", "36:20.0", "36:20.0", "36:20.1", "36:20.1", "36:20.1", "36:20.2", "36:20.2", "36:20.2", "36:20.3", "36:20.3", "36:20.3", "36:20.4", "36:20.4", "36:20.4", "36:20.5", "36:20.5", "36:20.5", "36:20.6", "36:20.6", "36:20.6", "36:20.7", "36:20.7", "36:20.7", "36:20.8", "36:20.8", "36:20.8", "36:20.9", "36:20.9", "36:20.9", "36:21.0", "36:21.0", "36:21.0", "36:21.1", "36:21.1", "36:21.1", "36:21.2", "36:21.2", "36:21.2", "36:21.3", "36:21.3", "36:21.3", "36:21.4", "36:21.4", "36:21.4", "36:21.5", "36:21.5", "36:21.5", "36:21.6", "36:21.6", "36:21.6", "36:21.7", "36:21.7", "36:21.7", "36:21.8", "36:21.8", "36:21.8", "36:21.9", "36:21.9", "36:21.9", "36:22.0", "36:22.0", "36:22.0", "36:22.1", "36:22.1", "36:22.1", "36:22.2", "36:22.2", "36:22.2", "36:22.3", "36:22.3", "36:22.3", "36:22.4", "36:22.4", "36:22.4", "36:22.5", "36:22.5", "36:22.5", "36:22.6", "36:22.6", "36:22.6", "36:22.7", "36:22.7", "36:22.7", "36:22.8", "36:22.8", "36:22.8", "36:22.9", "36:22.9", "36:22.9", "36:23.0", "36:23.0", "36:23.0", "36:23.1", "36:23.1", "36:23.1", "36:23.2", "36:23.2", "36:23.2", "36:23.3", "36:23.3", "36:23.3", "36:23.4", "36:23.4", "36:23.4", "36:23.5", "36:23.5", "36:23.5", "36:23.6", "36:23.6", "36:23.6", "36:23.7", "36:23.7", "36:23.7", "36:23.8", "36:23.8", "36:23.8", "36:23.9", "36:23.9", "36:23.9", "36:24.0", "36:24.0", "36:24.0", "36:24.1", "36:24.1", "36:24.1", "36:24.2", "36:24.2", "36:24.2", "36:24.3", "36:24.3", "36:24.3", "36:24.4", "36:24.4", "36:24.4", "36:24.5", "36:24.5", "36:24.5", "36:24.6", "36:24.6", "36:24.6", "36:24.7", "36:24.7", "36:24.7", "36:24.8", "36:24.8", "36:24.8", "36:24.9", "36:24.9", "36:24.9", "36:25.0", "36:25.0", "36:25.0", "36:25.1", "36:25.1", "36:25.1", "36:25.2", "36:25.2", "36:25.2", "36:25.3", "36:25.3", "36:25.3", "36:25.4", "36:25.4", "36:25.4", "36:25.5", "36:25.5", "36:25.5", "36:25.6", "36:25.6", "36:25.6", "36:25.7", "36:25.7", "36:25.7", "36:25.8", "36:25.8", "36:25.8", "36:25.9", "36:25.9", "36:25.9", "36:26.0", "36:26.0", "36:26.0", "36:26.1", "36:26.1", "36:26.1", "36:26.2", "36:26.2", "36:26.2", "36:26.3", "36:26.3", "36:26.3", "36:26.4", "36:26.4", "36:26.4", "36:26.5", "36:26.5", "36:26.5", "36:26.6", "36:26.6", "36:26.6", "36:26.7", "36:26.7", "36:26.7", "36:26.8", "36:26.8", "36:26.8", "36:26.9", "36:26.9", "36:26.9", "36:27.0", "36:27.0", "36:27.0", "36:27.1", "36:27.1", "36:27.1", "36:27.2", "36:27.2", "36:27.2", "36:27.3", "36:27.3", "36:27.3", "36:27.4", "36:27.4", "36:27.4", "36:27.5", "36:27.5", "36:27.5", "36:27.6", "36:27.6", "36:27.6", "36:27.7", "36:27.7", "36:27.7", "36:27.8", "36:27.8", "36:27.8", "36:27.9", "36:27.9", "36:27.9", "36:28.0", "36:28.0", "36:28.0", "36:28.1", "36:28.1", "36:28.1", "36:28.2", "36:28.2", "36:28.2", "36:28.3", "36:28.3", "36:28.3", "36:28.4", "36:28.4", "36:28.4", "36:28.5", "36:28.5", "36:28.5", "36:28.6", "36:28.6", "36:28.6", "36:28.7", "36:28.7", "36:28.7", "36:28.8", "36:28.8", "36:28.8", "36:28.9", "36:28.9", "36:28.9", "36:29.0", "36:29.0", "36:29.0", "36:29.1", "36:29.1", "36:29.1", "36:29.2", "36:29.2", "36:29.2", "36:29.3", "36:29.3", "36:29.3", "36:29.4", "36:29.4", "36:29.4", "36:29.5", "36:29.5", "36:29.5", "36:29.6", "36:29.6", "36:29.6", "36:29.7", "36:29.7", "36:29.7", "36:29.8", "36:29.8", "36:29.8", "36:29.9", "36:29.9", "36:29.9", "36:30.0", "36:30.0", "36:30.0", "36:30.1", "36:30.1", "36:30.1", "36:30.2", "36:30.2", "36:30.2", "36:30.3", "36:30.3", "36:30.3", "36:30.4", "36:30.4", "36:30.4", "36:30.5", "36:30.5", "36:30.5", "36:30.6", "36:30.6", "36:30.6", "36:30.7", "36:30.7", "36:30.7", "36:30.8", "36:30.8", "36:30.8", "36:30.9", "36:30.9", "36:30.9", "36:31.0", "36:31.0", "36:31.0", "36:31.1", "36:31.1", "36:31.1", "36:31.2", "36:31.2", "36:31.2", "36:31.3", "36:31.3", "36:31.3", "36:31.4", "36:31.4", "36:31.4", "36:31.5", "36:31.5", "36:31.5", "36:31.6", "36:31.6", "36:31.6", "36:31.7", "36:31.7", "36:31.7", "36:31.8", "36:31.8", "36:31.8", "36:31.9", "36:31.9", "36:31.9", "36:32.0", "36:32.0", "36:32.0", "36:32.1", "36:32.1", "36:32.1", "36:32.2", "36:32.2", "36:32.2", "36:32.3", "36:32.3", "36:32.3", "36:32.4", "36:32.4", "36:32.4", "36:32.5", "36:32.5", "36:32.5", "36:32.6", "36:32.6", "36:32.6", "36:32.7", "36:32.7", "36:32.7", "36:32.8", "36:32.8", "36:32.8", "36:32.9", "36:32.9", "36:32.9", "36:33.0", "36:33.0", "36:33.0", "36:33.1", "36:33.1", "36:33.1", "36:33.2", "36:33.2", "36:33.2", "36:33.3", "36:33.3", "36:33.3", "36:33.4", "36:33.4", "36:33.4", "36:33.5", "36:33.5", "36:33.5", "36:33.6", "36:33.6", "36:33.6", "36:33.7", "36:33.7", "36:33.7", "36:33.8", "36:33.8", "36:33.8", "36:33.9", "36:33.9", "36:33.9", "36:34.0", "36:34.0", "36:34.0", "36:34.1", "36:34.1", "36:34.1", "36:34.2", "36:34.2", "36:34.2", "36:34.3", "36:34.3", "36:34.3", "36:34.4", "36:34.4", "36:34.4", "36:34.5", "36:34.5", "36:34.5", "36:34.6", "36:34.6", "36:34.6", "36:34.7", "36:34.7", "36:34.7", "36:34.8", "36:34.8", "36:34.8", "36:34.9", "36:34.9", "36:34.9", "36:35.0", "36:35.0", "36:35.0", "36:35.1", "36:35.1", "36:35.1", "36:35.2", "36:35.2", "36:35.2", "36:35.3", "36:35.3", "36:35.3", "36:35.4", "36:35.4", "36:35.4", "36:35.5", "36:35.5", "36:35.5", "36:35.6", "36:35.6", "36:35.6", "36:35.7", "36:35.7", "36:35.7", "36:35.8", "36:35.8", "36:35.8", "36:35.9", "36:35.9", "36:35.9", "36:36.0", "36:36.0", "36:36.0", "36:36.1", "36:36.1", "36:36.1", "36:36.2", "36:36.2", "36:36.2", "36:36.3", "36:36.3", "36:36.3", "36:36.4", "36:36.4", "36:36.4", "36:36.5", "36:36.5", "36:36.5", "36:36.6", "36:36.6", "36:36.6", "36:36.7", "36:36.7", "36:36.7", "36:36.8", "36:36.8", "36:36.8", "36:36.9", "36:36.9", "36:36.9", "36:37.0", "36:37.0", "36:37.0", "36:37.1", "36:37.1", "36:37.1", "36:37.2", "36:37.2", "36:37.2", "36:37.3", "36:37.3", "36:37.3", "36:37.4", "36:37.4", "36:37.4", "36:37.5", "36:37.5", "36:37.5", "36:37.6", "36:37.6", "36:37.6", "36:37.7", "36:37.7", "36:37.7", "36:37.8", "36:37.8", "36:37.8", "36:37.9", "36:37.9", "36:37.9", "36:38.0", "36:38.0", "36:38.0", "36:38.1", "36:38.1", "36:38.1", "36:38.2", "36:38.2", "36:38.2", "36:38.3", "36:38.3", "36:38.3", "36:38.4", "36:38.4", "36:38.4", "36:38.5", "36:38.5", "36:38.5", "36:38.6", "36:38.6", "36:38.6", "36:38.7", "36:38.7", "36:38.7", "36:38.8", "36:38.8", "36:38.8", "36:38.9", "36:38.9", "36:38.9", "36:39.0", "36:39.0", "36:39.0", "36:39.1", "36:39.1", "36:39.1", "36:39.2", "36:39.2", "36:39.2", "36:39.3", "36:39.3", "36:39.3", "36:39.4", "36:39.4", "36:39.4", "36:39.5", "36:39.5", "36:39.5", "36:39.6", "36:39.6", "36:39.6", "36:39.7", "36:39.7", "36:39.7", "36:39.8", "36:39.8", "36:39.8", "36:39.9", "36:39.9", "36:39.9", "36:40.0", "36:40.0", "36:40.0", "36:40.1", "36:40.1", "36:40.1", "36:40.2", "36:40.2", "36:40.2", "36:40.3", "36:40.3", "36:40.3", "36:40.4", "36:40.4", "36:40.4", "36:40.5", "36:40.5", "36:40.5", "36:40.6", "36:40.6", "36:40.6", "36:40.7", "36:40.7", "36:40.7", "36:40.8", "36:40.8", "36:40.8", "36:40.9", "36:40.9", "36:40.9", "36:41.0", "36:41.0", "36:41.0", "36:41.1", "36:41.1", "36:41.1", "36:41.2", "36:41.2", "36:41.2", "36:41.3", "36:41.3", "36:41.3", "36:41.4", "36:41.4", "36:41.4", "36:41.5", "36:41.5", "36:41.5", "36:41.6", "36:41.6", "36:41.6", "36:41.7", "36:41.7", "36:41.7", "36:41.8", "36:41.8", "36:41.8", "36:41.9", "36:41.9", "36:41.9", "36:42.0", "36:42.0", "36:42.0", "36:42.1", "36:42.1", "36:42.1", "36:42.2", "36:42.2", "36:42.2", "36:42.3", "36:42.3", "36:42.3", "36:42.4", "36:42.4", "36:42.4", "36:42.5", "36:42.5", "36:42.5", "36:42.6", "36:42.6", "36:42.6", "36:42.7", "36:42.7", "36:42.7", "36:42.8", "36:42.8", "36:42.8", "36:42.9", "36:42.9", "36:42.9", "36:43.0", "36:43.0", "36:43.0", "36:43.1", "36:43.1", "36:43.1", "36:43.2", "36:43.2", "36:43.2", "36:43.3", "36:43.3", "36:43.3", "36:43.4", "36:43.4", "36:43.4", "36:43.5", "36:43.5", "36:43.5", "36:43.6", "36:43.6", "36:43.6", "36:43.7", "36:43.7", "36:43.7", "36:43.8", "36:43.8", "36:43.8", "36:43.9", "36:43.9", "36:43.9", "36:44.0", "36:44.0", "36:44.0", "36:44.1", "36:44.1", "36:44.1", "36:44.2", "36:44.2", "36:44.2", "36:44.3", "36:44.3", "36:44.3", "36:44.4", "36:44.4", "36:44.4", "36:44.5", "36:44.5", "36:44.5", 
